vi "Calc Cmd Numeric.vi"(8 "error in (no error)":errorcluster, 9 "Cmd Value":dbl, 10 "Name":string, 11 "Calculation in":refnum<class "Calculation.lvclass">) -> (0 "error out":errorcluster, 3 "Calculation out":refnum<class "Calculation.lvclass">)   [LabVIEW 2020, in "VolatusCalcs.lvlib" / "Calculation.lvclass"]
uses:
  Calculation.lvclass
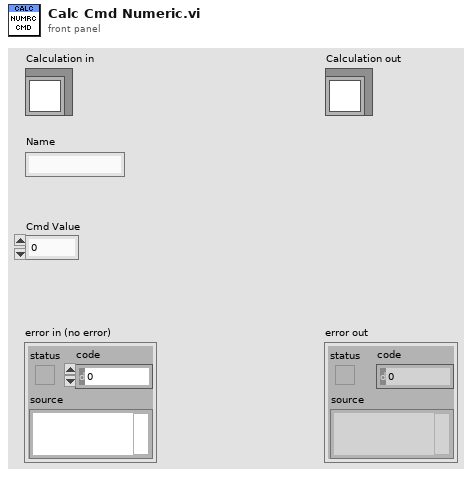
[diagram p1: front panel]
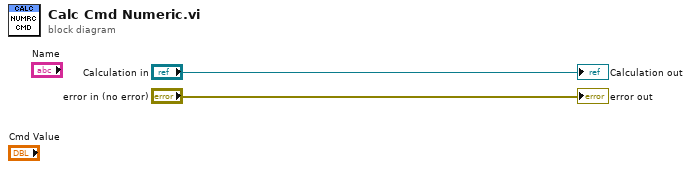
[diagram p0: block diagram]
diagram:
  "error out" <- "error in (no error)"
  "Calculation out" <- "Calculation in"
